vi "Recursion_Hanoi_E.vi"(8 "C":string="C", 9 "B":string="B", 10 "A":string="A", 11 "Plates":u8=4) -> (3 "Step":string[](array[string]))   [LabVIEW 2012]
panel:
  out "Total_stp":i32
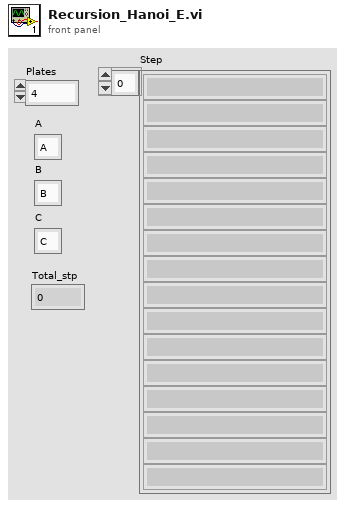
[diagram p1: front panel]
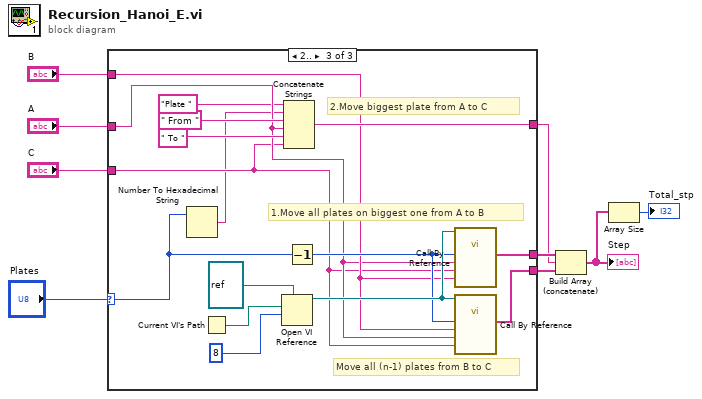
[diagram p0: block diagram]
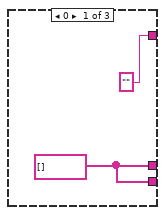
[diagram p2: hidden frame]
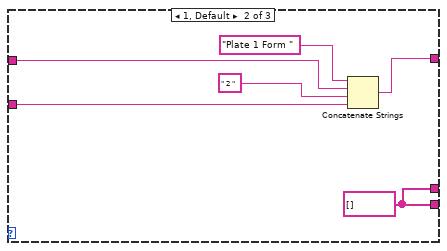
[diagram p3: hidden frame]
diagram:
  n1 = case shown="2.." "Plates" {
    selector: "Plates" -> [_ _ w20]
    tunnel: [w11 w17 w31] -> w8
    tunnel: ["" w12 w28] -> w7
    tunnel: "A" -> [_ w15 w23]
    tunnel: "C" -> [_ w13 w22]
    tunnel: [w11 w17 w25] -> w4
    tunnel: "B" -> [_ _ w24]
    frame 0 {
      w11 = string[] [] ("Array")
    }
    frame 1, Default {
      w17 = string[] [] ("Array")
      n2 = Concatenate Strings("Plate 1 Form ", w15, " 2 ", w13) -> (w12:string)
    }
    frame 2.. {
      # "2.Move biggest plate from A to C"
      # "Move all (n-1) plates from B to C"
      # "1.Move all plates on biggest one from A to B"
      n3 = Number To Hexadecimal String(2:w20) -> (0:w18:string)  [unwired: 1 in]
      n4 = Current VI's Path() -> (path=w21:path)
      n5 = Open VI Reference(type specifier VI Refnum (for type only)=refnum<vi> refnum, vi path=w21, options=8) -> (vi reference=w27:refnum<vi>)  [unwired: 3 in, 1 out]
      n6 = Concatenate Strings("Plate ", w18, " From ", w23, " To ", w22) -> (w28:string)
      n7 = Decrement(x=w20) -> (x-1=w26:u8)
      n8 = call-by-ref "?"(reference=w27, "C"=w24, "B"=w22, "A"=w23, "x (input)"=w26) -> ("Array"=w31:string[])  [unwired: 8 in, 2 out]
      n9 = call-by-ref "?"(reference=w27, "C"=w22, "B"=w23, "A"=w24, "x (input)"=w26) -> ("Array"=w25:string[])  [unwired: 8 in, 2 out]
    }
  }
  n10 = Build Array (concatenate)(w8, w7, w4) -> (w2:string[])
  "Step" <- w2
  n11 = Array Size(array=w2) -> (size(s)=→"Total_stp":i32)
